vi "From JSON Text (timestamp).vi"(7 "Data Type (default value)":timestamp, 9 "error in (no error)":errorcluster, 10 "Offset":i32, 11 "JSON":string) -> (1 "error out":errorcluster, 2 "Offset past match":i32, 3 "Time Stamp":timestamp)   [LabVIEW 2015, in "JSONtext.lvlib"]
doc: "Convert the JSON Value at Offset into a LabVIEW type."
uses:
  JSONtext.lvlib
  Get Timestamp.vi
  Advance past whitespace.vi
  Format Error.vi
  Get String.vi
  Get U64.vi
  Advance past String.vi
  String Subset.vi
  support/Strip Quotes and Unescape.vi
  Get Number Text.vi
  NaN or null to Integer ERROR.vi
  Advance past Number.vi
  <vilib>/Utility/error.llb/Error Cluster From Error Code.vi
  Parsing Error.vi
  support/Scan Timestamp.vi
  support/Unescape JSON string.vi
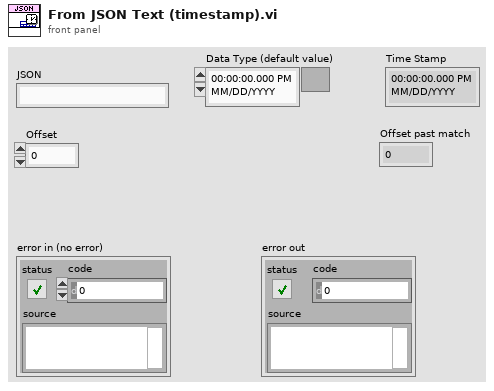
[diagram p1: front panel]
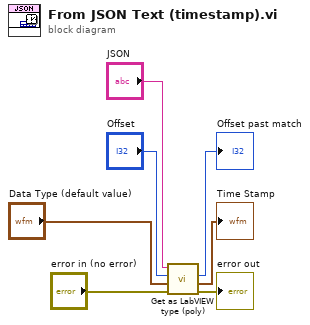
[diagram p0: block diagram]
diagram:
  n1 = call-poly "Get as LabVIEW type (poly).vi"("error in (no error)"="error in (no error)", "Data Type (default value)"="Data Type (default value)", "Offset"="Offset", "JSON"="JSON") -> ("error out"=→"error out":errorcluster, "Timestamp"=→"Time Stamp":timestamp, "Offset past match"=→"Offset past match":i32)  [unwired: 5 in]
